vi "Prova NPSH.vi"(7 "Tipo motore pompa":enum16{"Monofase", "Trifase"}(ring), 8 "Array % valvole":dbl[][](array[numeric]), 9 "Manuale F\\auto T":bool=TRUE, 11 "input cluster":T1={"Coefficenti P2"={"Af"=0.0, "Bf"=0.0, "Cf"=0.0, "Df"=0.0, "Ef"=0.0, "Ff"=0.0, "Gf"=0.0, "Hf"=0.0, "Jf"=0.0, "Kf"=0.0, "If"=0.0, "Ar"=0.0, "Br"=0.0, "Cr"=0.0, "Dr"=0.0, "Er"=0.0, "Fr"=0.0, "Gr"=0.0, "Hr"=0.0, "Jr"=0.0, "Kr"=0.0, "Ir"=0.0}, "Cluster settaggi wattmetro"={"Wattmetro"=enum."WT230", "Alimentazione"=enum."Radio Selection 1"}, "CALCOLO POTENZA MECCANICA?"=FALSE, "SET RPM"=0.0, "SET TEMP"=0.0, "IMPOSTAZIONI INGRESSI UL"={"SALVA"=FALSE, "CARICA"=FALSE, "APPLICA"=FALSE, "Q1"={"Range"=0.0, "Offset"=0.0, "Medie"=0}, "Q2"={"Range"=0.0, "Offset"=0.0, "Medie"=0}, "Q3"={"Range"=0.0, "Offset"=0.0, "Medie"=0}, "P1"={"Range"=0.0, "Offset"=0.0, "Medie"=0}, "P2"={"Range"=0.0, "Offset"=0.0, "Medie"=0}, "P3"={"Range"=0.0, "Offset"=0.0, "Medie"=0}, "N"={"Range"=0.0, "Offset"=0.0, "Medie"=0}, "Tq"={"Range"=0.0, "Offset"=0.0, "Medie"=0}, "T"={"Range"=0.0, "Offset"=0.0, "Medie"=0}, "PORTATA PRINCIPALE"=0, "PORTATA SECONDARIA"=0, "PRESSIONE ASPIRAZIONE"=0, "PRESSIONE MANDATA"=0, "RPM"=0, "differenziale?"=FALSE}, "IMPOSTAZIONI INGRESSI NM"={"SALVA"=FALSE, "CARICA"=FALSE, "APPLICA"=FALSE, "Q1"={"Range"=0.0, "Offset"=0.0, "Medie"=0}, "Q2"={"Range"=0.0, "Offset"=0.0, "Medie"=0}, "Q3"={"Range"=0.0, "Offset"=0.0, "Medie"=0}, "Q4"={"Range"=0.0, "Offset"=0.0, "Medie"=0}, "Q5"={"Range"=0.0, "Offset"=0.0, "Medie"=0}, "Q6"={"Range"=0.0, "Offset"=0.0, "Medie"=0}, "Q7"={"Range"=0.0, "Offset"=0.0, "Medie"=0}, "Q8"={"Range"=0.0, "Offset"=0.0, "Medie"=0}, "Q9"={"Range"=0.0, "Offset"=0.0, "Medie"=0}, "Q10"={"Range"=0.0, "Offset"=0.0, "Medie"=0}, "P1"={"Range"=0.0, "Offset"=0.0, "Medie"=0}, "P2"={"Range"=0.0, "Offset"=0.0, "Medie"=0}, "P3"={"Range"=0.0, "Offset"=0.0, "Medie"=0}, "P4"={"Range"=0.0, "Offset"=0.0, "Medie"=0}, "P5"={"Range"=0.0, "Offset"=0.0, "Medie"=0}, "P6"={"Range"=0.0, "Offset"=0.0, "Medie"=0}, "P7"={"Range"=0.0, "Offset"=0.0, "Medie"=0}, "P8"={"Range"=0.0, "Offset"=0.0, "Medie"=0}, "P9"={"Range"=0.0, "Offset"=0.0, "Medie"=0}, "P10"={"Range"=0.0, "Offset"=0.0, "Medie"=0}, "N1(T)"={"Range"=0.0, "Offset"=0.0, "Medie"=0}, "N2(T)"={"Range"=0.0, "Offset"=0.0, "Medie"=0}, "N3(T)"={"Range"=0.0, "Offset"=0.0, "Medie"=0}, "Tq1"={"Range"=0.0, "Offset"=0.0, "Medie"=0}, "Tq2"={"Range"=0.0, "Offset"=0.0, "Medie"=0}, "Tq3"={"Range"=0.0, "Offset"=0.0, "Medie"=0}, "RM1"={"Range"=0.0, "Offset"=0.0, "Medie"=0}, "RM2"={"Range"=0.0, "Offset"=0.0, "Medie"=0}, "RM3"={"Range"=0.0, "Offset"=0.0, "Medie"=0}, "T1"={"Range"=0.0, "Offset"=0.0, "Medie"=0}, "T2"={"Range"=0.0, "Offset"=0.0, "Medie"=0}, "T3"={"Range"=0.0, "Offset"=0.0, "Medie"=0}, "T4"={"Range"=0.0, "Offset"=0.0, "Medie"=0}, "T5"={"Range"=0.0, "Offset"=0.0, "Medie"=0}, "T6"={"Range"=0.0, "Offset"=0.0, "Medie"=0}, "T7"={"Range"=0.0, "Offset"=0.0, "Medie"=0}, "T8"={"Range"=0.0, "Offset"=0.0, "Medie"=0}, "Liv."={"Range"=0.0, "Offset"=0.0, "Medie"=0}, "Pbar"={"Range"=0.0, "Offset"=0.0, "Medie"=0}, "PORTATA\nPRINCIPALE"=0, "PORTATA\nSECONDARIA"=0, "PRESSIONE\nASPIRAZIONE"=0, "PRESSIONE\nMANDATA"=0, "RPM"=0, "differenziale?"=FALSE}, "Costanti collaudo"={"P [bar]"=0.0, "T amb. [°C]"=0.0, "Umidità [%]"=0.0}, "Condizione P2"=enum."Radio Selection 1", "Sett T e R"={"Tamb[°C]"=0.0, "Ru-w"=0.0, "Rmarcia"=0.0, "Raux"=0.0, "Ru-w freddo"=0.0, "Rmarcia freddo"=0.0, "Raux freddop"=0.0, "TC1"=0.0, "TC2"=0.0, "TC3"=0.0, "TC4"=0.0, "TC5"=0.0, "TC6"=0.0, "TC7"=0.0, "TC8"=0.0, "TC9"=0.0}, "Array linee"=[{"portata"=0, "Hasp"=0, "Hmand"=1, "Torsiometro"=0, "rpm"=0, "Hdiff?"=FALSE, "T amb"=0, "Indici valvole"=[0, 1], "Nome"="Elettropompa", "Sommersa?"=FALSE}, {"portata"=1, "Hasp"=0, "Hmand"=0, "Torsiometro"=0, "rpm"=0, "Hdiff?"=FALSE, "T amb"=0, "Indici valvole"=[0, 1], "Nome"="Sommersa", "Sommersa?"=TRUE}], "Array valvole linee avvio/fermata"=[], "Linea selezionata"=0.0} {"IMPOSTAZIONI INGRESSI NM"."T8"."Medie" min=1 step=1; "IMPOSTAZIONI INGRESSI NM"."T7"."Medie" min=1 step=1; "IMPOSTAZIONI INGRESSI NM"."T6"."Medie" min=1 step=1; "IMPOSTAZIONI INGRESSI NM"."T5"."Medie" min=1 step=1; "IMPOSTAZIONI INGRESSI NM"."T4"."Medie" min=1 step=1; "IMPOSTAZIONI INGRESSI NM"."T3"."Medie" min=1 step=1; "IMPOSTAZIONI INGRESSI NM"."RM3"."Medie" min=1 step=1; "IMPOSTAZIONI INGRESSI NM"."Tq3"."Medie" min=1 step=1; "IMPOSTAZIONI INGRESSI NM"."Tq2"."Medie" min=1 step=1; "IMPOSTAZIONI INGRESSI NM"."N3(T)"."Medie" min=1 step=1; "IMPOSTAZIONI INGRESSI NM"."N2(T)"."Medie" min=1 step=1; "IMPOSTAZIONI INGRESSI NM"."P10"."Medie" min=1 step=1; "IMPOSTAZIONI INGRESSI NM"."P9"."Medie" min=1 step=1; "IMPOSTAZIONI INGRESSI NM"."P8"."Medie" min=1 step=1; "IMPOSTAZIONI INGRESSI NM"."P7"."Medie" min=1 step=1; "IMPOSTAZIONI INGRESSI NM"."P6"."Medie" min=1 step=1; "IMPOSTAZIONI INGRESSI NM"."P5"."Medie" min=1 step=1; "IMPOSTAZIONI INGRESSI NM"."Q10"."Medie" min=1 step=1; "IMPOSTAZIONI INGRESSI NM"."Q9"."Medie" min=1 step=1; "IMPOSTAZIONI INGRESSI NM"."Q8"."Medie" min=1 step=1; "IMPOSTAZIONI INGRESSI NM"."Q7"."Medie" min=1 step=1; "IMPOSTAZIONI INGRESSI NM"."Q6"."Medie" min=1 step=1; "IMPOSTAZIONI INGRESSI NM"."Q5"."Medie" min=1 step=1; "IMPOSTAZIONI INGRESSI NM"."Pbar"."Medie" min=1 step=1; "IMPOSTAZIONI INGRESSI NM"."Liv."."Medie" min=1 step=1; "IMPOSTAZIONI INGRESSI NM"."RM2"."Medie" min=1 step=1; "IMPOSTAZIONI INGRESSI NM"."RM1"."Medie" min=1 step=1; "IMPOSTAZIONI INGRESSI NM"."T2"."Medie" min=1 step=1; "IMPOSTAZIONI INGRESSI NM"."P4"."Medie" min=1 step=1; "IMPOSTAZIONI INGRESSI NM"."Q4"."Medie" min=1 step=1; "IMPOSTAZIONI INGRESSI NM"."RPM" items=["TESTO", "TORSIOMETRO", "OTTICA"]; "IMPOSTAZIONI INGRESSI NM"."PRESSIONE\nMANDATA" items=["P1", "P2", "P3", "P4"]; "IMPOSTAZIONI INGRESSI NM"."PRESSIONE\nASPIRAZIONE" items=["P1", "P2", "P3", "P4"]; "IMPOSTAZIONI INGRESSI NM"."PORTATA\nSECONDARIA" items=["Q1", "Q2", "Q3", "Q4"]; "IMPOSTAZIONI INGRESSI NM"."PORTATA\nPRINCIPALE" items=["LINEA ELETTROPOMPA", "LINEA SOMMERSA"]; "IMPOSTAZIONI INGRESSI NM"."T1"."Medie" min=1 step=1; "IMPOSTAZIONI INGRESSI NM"."Tq1"."Medie" min=1 step=1; "IMPOSTAZIONI INGRESSI NM"."N1(T)"."Medie" min=1 step=1; "IMPOSTAZIONI INGRESSI NM"."P3"."Medie" min=1 step=1; "IMPOSTAZIONI INGRESSI NM"."P2"."Medie" min=1 step=1; "IMPOSTAZIONI INGRESSI NM"."P1"."Medie" min=1 step=1; "IMPOSTAZIONI INGRESSI NM"."Q3"."Medie" min=1 step=1; "IMPOSTAZIONI INGRESSI NM"."Q2"."Medie" min=1 step=1; "IMPOSTAZIONI INGRESSI NM"."Q1"."Medie" min=1 step=1; "IMPOSTAZIONI INGRESSI UL"."RPM" items=["TESTO", "TORSIOMETRO", "OTTICA"]; "IMPOSTAZIONI INGRESSI UL"."PRESSIONE MANDATA" items=["P1", "P2", "P3"]; "IMPOSTAZIONI INGRESSI UL"."PRESSIONE ASPIRAZIONE" items=["P1", "P2", "P3"]; "IMPOSTAZIONI INGRESSI UL"."PORTATA SECONDARIA" items=["Q1", "Q2", "Q3"]; "IMPOSTAZIONI INGRESSI UL"."PORTATA PRINCIPALE" items=["Q1", "Q2", "Q3"]; "IMPOSTAZIONI INGRESSI UL"."T"."Medie" min=1 step=1; "IMPOSTAZIONI INGRESSI UL"."Tq"."Medie" min=1 step=1; "IMPOSTAZIONI INGRESSI UL"."N"."Medie" min=1 step=1; "IMPOSTAZIONI INGRESSI UL"."P3"."Medie" min=1 step=1; "IMPOSTAZIONI INGRESSI UL"."P2"."Medie" min=1 step=1; "IMPOSTAZIONI INGRESSI UL"."P1"."Medie" min=1 step=1; "IMPOSTAZIONI INGRESSI UL"."Q3"."Medie" min=1 step=1; "IMPOSTAZIONI INGRESSI UL"."Q2"."Medie" min=1 step=1; "IMPOSTAZIONI INGRESSI UL"."Q1"."Medie" min=1 step=1}) -> ()   [LabVIEW 2016]
uses:
  TypeDef/ALIM SELECTION.ctl
  TypeDef/WT SELECTION.ctl
  TypeDef/SETUP INGRESSO.ctl
  TypeDef/cDAQ Settings UL.ctl
  TypeDef/cDAQ Settings NM.ctl
  TypeDef/sett T e R.ctl
  TypeDef/Definizione linea.ctl
  TypeDef/Cluster INFO.ctl
panel:
  in  "Status":refnum<vi>
  # "Freddo"
  # "Regime"
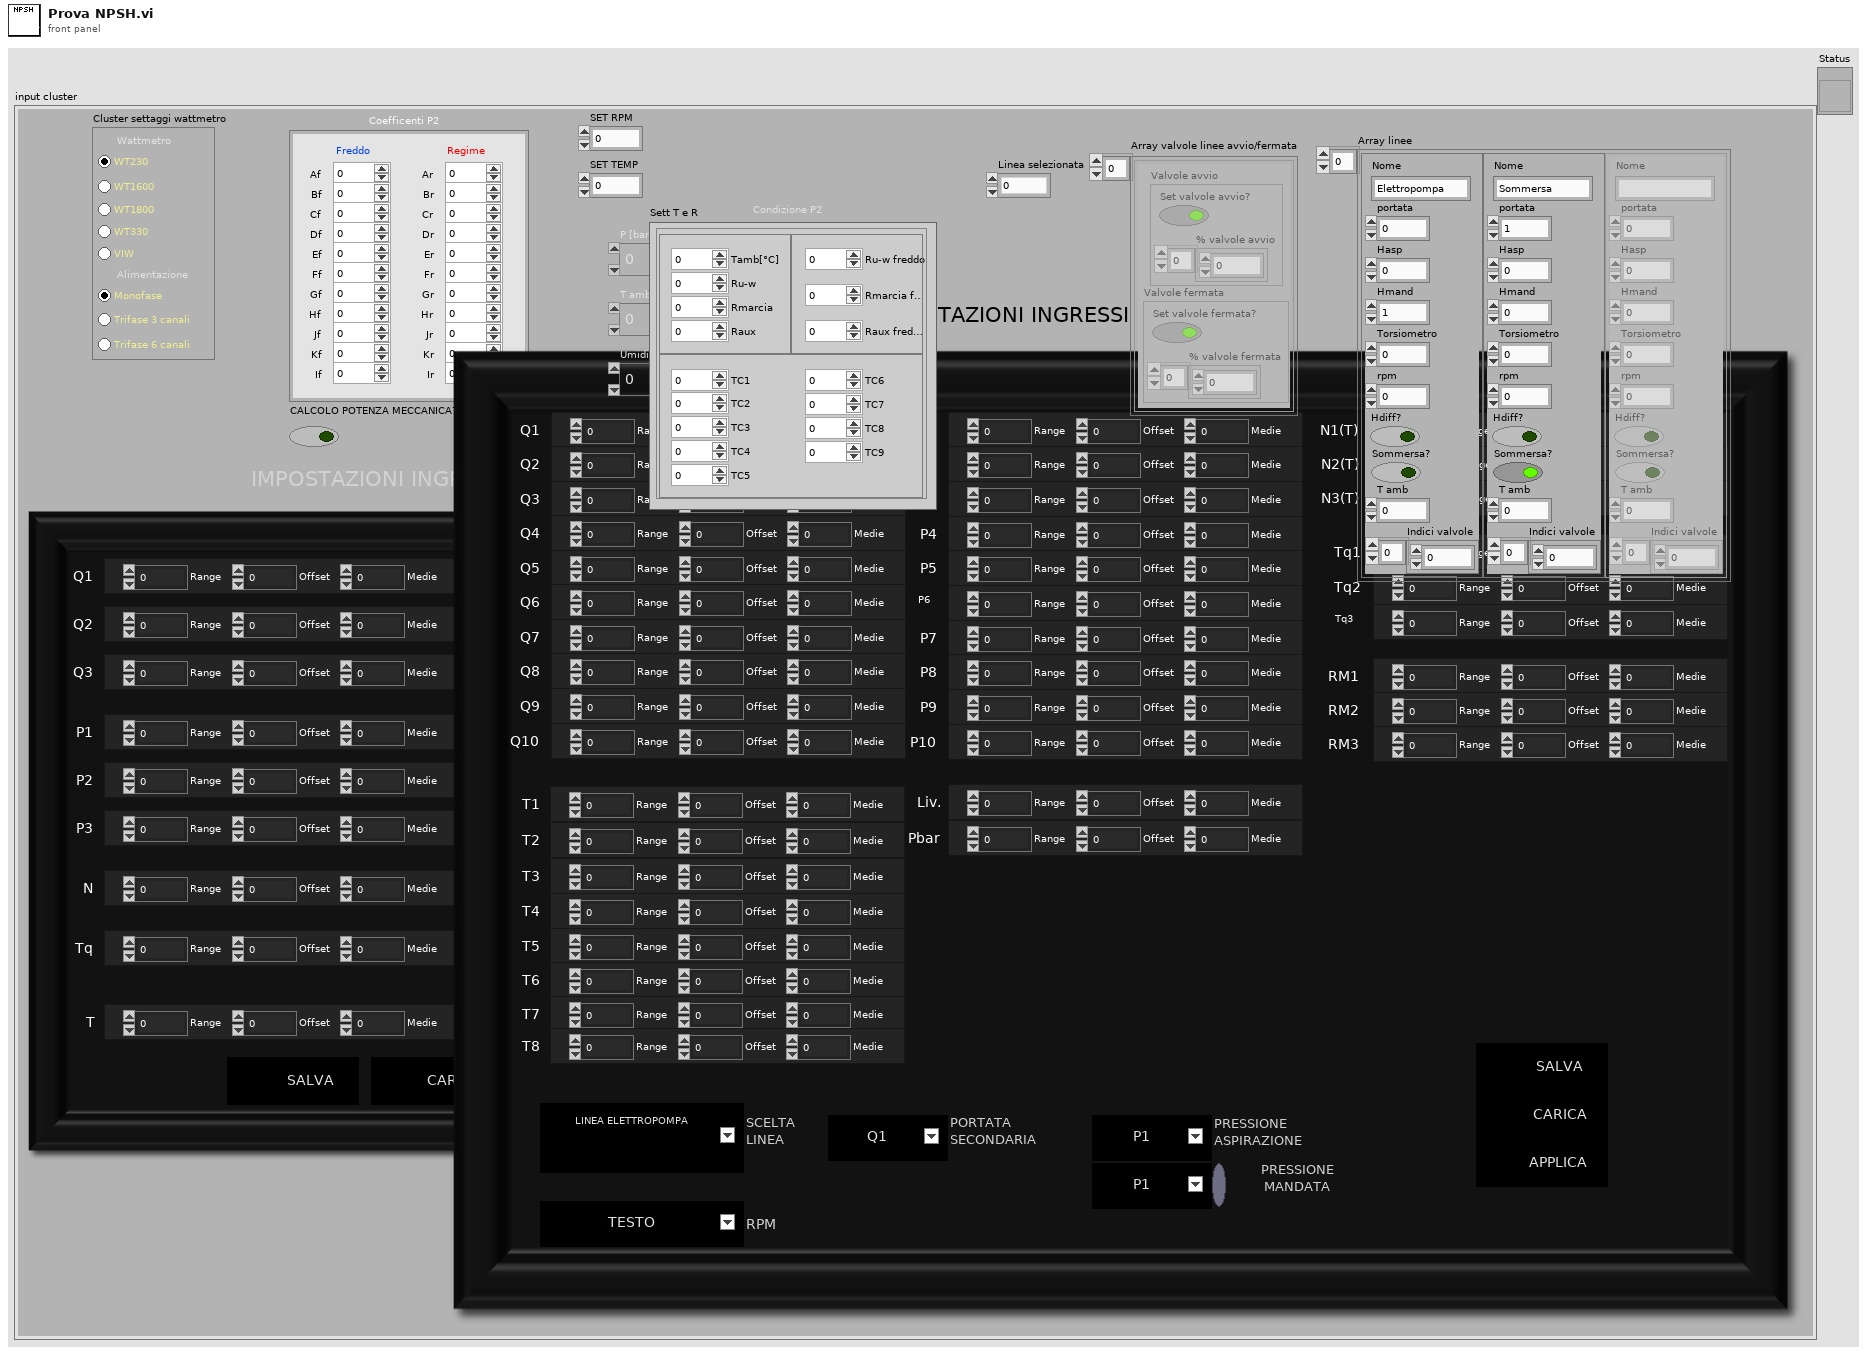
[diagram p1: front panel]
types:
  T1 = typedef "Cluster INFO.ctl" = cluster{"Coefficenti P2":cluster{"Af":dbl, "Bf":dbl, "Cf":dbl, "Df":dbl, "Ef":dbl, "Ff":dbl, "Gf":dbl, "Hf":dbl, "Jf":dbl, "Kf":dbl, "If":dbl, "Ar":dbl, "Br":dbl, "Cr":dbl, "Dr":dbl, "Er":dbl, "Fr":dbl, "Gr":dbl, "Hr":dbl, "Jr":dbl, "Kr":dbl, "Ir":dbl}, "Cluster settaggi wattmetro":cluster{"Wattmetro":T2, "Alimentazione":T3}, "CALCOLO POTENZA MECCANICA?":bool, "SET RPM":dbl, "SET TEMP":dbl, "IMPOSTAZIONI INGRESSI UL":T4, "IMPOSTAZIONI INGRESSI NM":T6, "Costanti collaudo":cluster{"P [bar]":dbl, "T amb. [°C]":dbl, "Umidità [%]":dbl}, "Condizione P2":enum32{"Radio Selection 1", "Radio Selection 2"}, "Sett T e R":T7, "Array linee":T8[], "Array valvole linee avvio/fermata":cluster{"Valvole avvio":cluster{"Set valvole avvio?":bool, "% valvole avvio":dbl[]}, "Valvole fermata":cluster{"Set valvole fermata?":bool, "% valvole fermata":dbl[]}}[], "Linea selezionata":dbl}
  T2 = typedef "WT SELECTION.ctl" = enum32{"No Selection", "WT230", "WT1600", "WT1800", "WT330", "VIW"}
  T3 = typedef "ALIM SELECTION.ctl" = enum32{"Radio Selection 1", "Radio Selection 2", "Radio Selection 3"}
  T4 = typedef "cDAQ Settings UL.ctl" = cluster{"SALVA":bool, "CARICA":bool, "APPLICA":bool, "Q1":T5, "Q2":T5, "Q3":T5, "P1":T5, "P2":T5, "P3":T5, "N":T5, "Tq":T5, "T":T5, "PORTATA PRINCIPALE":u16, "PORTATA SECONDARIA":u16, "PRESSIONE ASPIRAZIONE":u16, "PRESSIONE MANDATA":u16, "RPM":u16, "differenziale?":bool}
  T5 = typedef "SETUP INGRESSO.ctl" = cluster{"Range":dbl, "Offset":dbl, "Medie":u8}
  T6 = typedef "cDAQ Settings NM.ctl" = cluster{"SALVA":bool, "CARICA":bool, "APPLICA":bool, "Q1":T5, "Q2":T5, "Q3":T5, "Q4":T5, "Q5":T5, "Q6":T5, "Q7":T5, "Q8":T5, "Q9":T5, "Q10":T5, "P1":T5, "P2":T5, "P3":T5, "P4":T5, "P5":T5, "P6":T5, "P7":T5, "P8":T5, "P9":T5, "P10":T5, "N1(T)":T5, "N2(T)":T5, "N3(T)":T5, "Tq1":T5, "Tq2":T5, "Tq3":T5, "RM1":T5, "RM2":T5, "RM3":T5, "T1":T5, "T2":T5, "T3":T5, "T4":T5, "T5":T5, "T6":T5, "T7":T5, "T8":T5, "Liv.":T5, "Pbar":T5, "PORTATA\nPRINCIPALE":u16, "PORTATA\nSECONDARIA":u16, "PRESSIONE\nASPIRAZIONE":u16, "PRESSIONE\nMANDATA":u16, "RPM":u16, "differenziale?":bool}
  T7 = typedef "sett T e R.ctl" = cluster{"Tamb[°C]":dbl, "Ru-w":dbl, "Rmarcia":dbl, "Raux":dbl, "Ru-w freddo":dbl, "Rmarcia freddo":dbl, "Raux freddop":dbl, "TC1":dbl, "TC2":dbl, "TC3":dbl, "TC4":dbl, "TC5":dbl, "TC6":dbl, "TC7":dbl, "TC8":dbl, "TC9":dbl}
  T8 = typedef "Definizione linea.ctl" = cluster{"portata":i32, "Hasp":i32, "Hmand":i32, "Torsiometro":i32, "rpm":i32, "Hdiff?":bool, "T amb":i32, "Indici valvole":i16[], "Nome":string, "Sommersa?":bool}
  T9 = cluster{"Valvole avvio":cluster{"Set valvole avvio?":bool, "% valvole avvio":dbl[]}, "Valvole fermata":cluster{"Set valvole fermata?":bool, "% valvole fermata":dbl[]}}[]
  T10 = cluster{"Valvole avvio":cluster{"Set valvole avvio?":bool, "% valvole avvio":dbl[]}, "Valvole fermata":cluster{"Set valvole fermata?":bool, "% valvole fermata":dbl[]}}
  T11 = cluster{"Set valvole avvio?":bool, "% valvole avvio":dbl[]}
  T12 = cluster{"Set valvole fermata?":bool, "% valvole fermata":dbl[]}
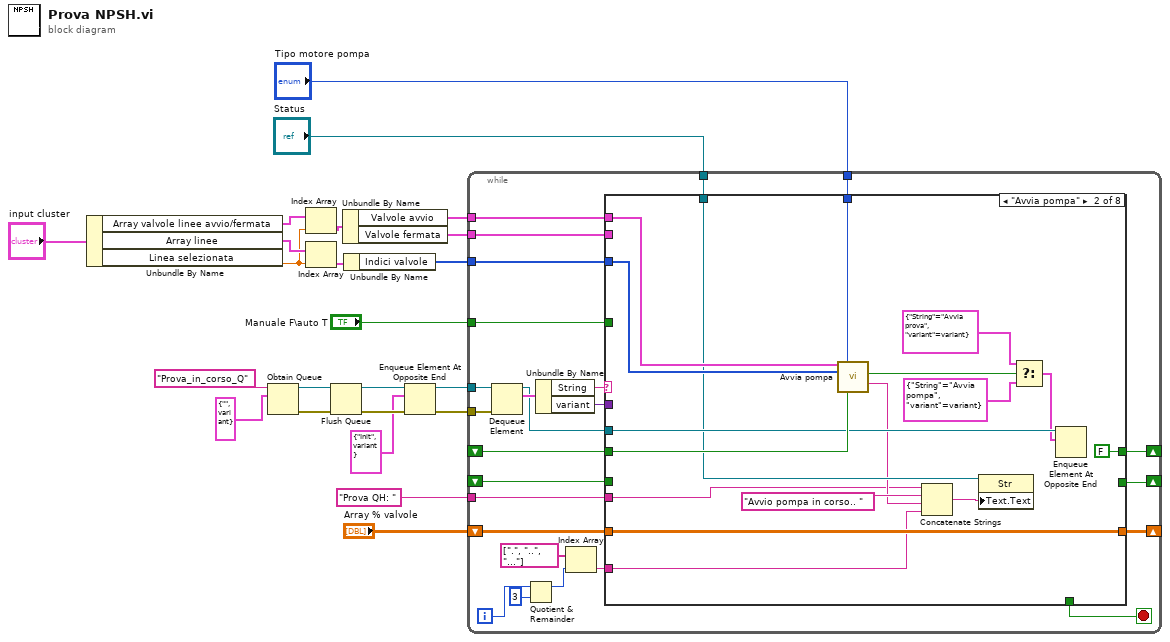
[diagram p0: block diagram]
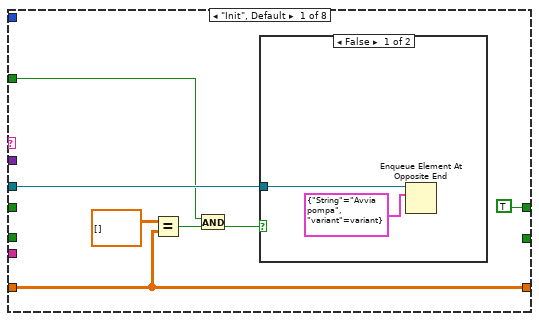
[diagram p2: hidden frame]
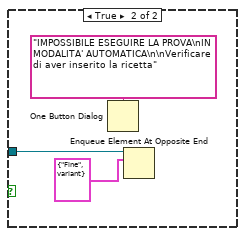
[diagram p3: hidden frame]
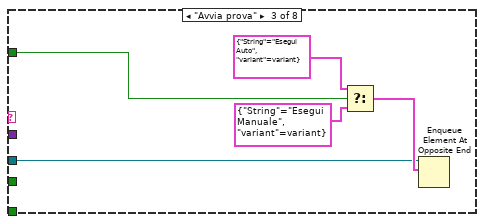
[diagram p4: hidden frame]
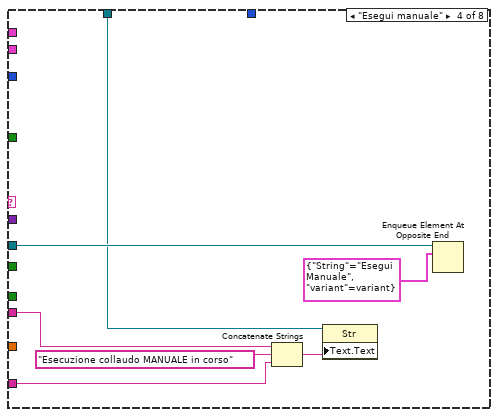
[diagram p5: hidden frame]
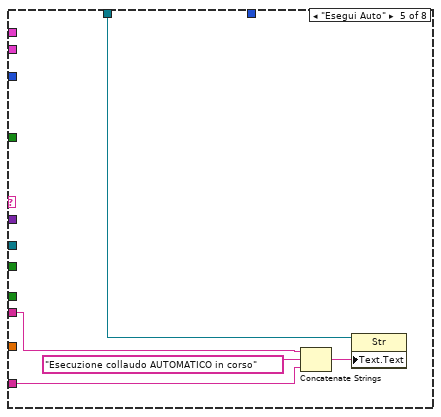
[diagram p6: hidden frame]
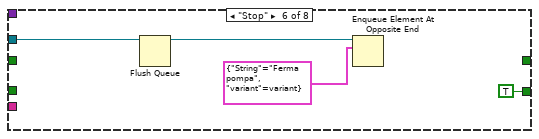
[diagram p7: hidden frame]
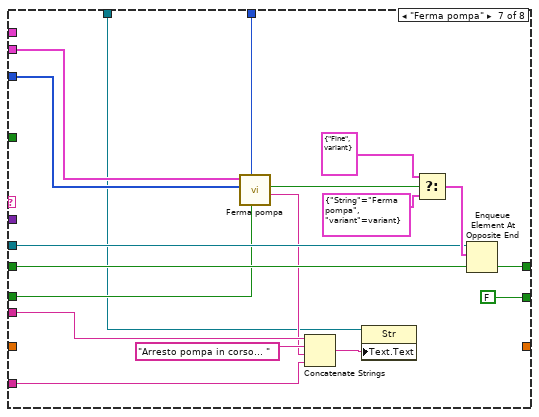
[diagram p8: hidden frame]
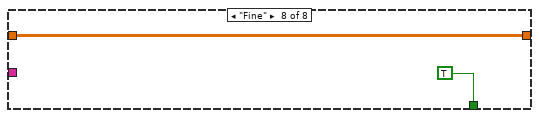
[diagram p9: hidden frame]
diagram:
  n1 = Unbundle By Name("input cluster") -> ("Array valvole linee avvio/fermata"=w9:T9, "Array linee"=w11:T8[], "Linea selezionata"=w8:dbl)
  n2 = Obtain Queue(name (unnamed)="Prova_in_corso_Q" ("Queue Name"), element data type=cluster{"String":string, "variant":variant} {"String"="", "variant"=variant} ("element")) -> (queue out=w17:refnum<queue>, error out=w16:errorcluster)  [unwired: 3 in, 1 out]
  n3 = Index Array(array=w9, index=w8) -> (element=w7:T10)
  n4 = Index Array(array=w11, index=w8) -> (element=w10:T8)
  n5 = Flush Queue(queue=w17, error in (no error)=w16) -> (queue out=w21:refnum<queue>, error out=w20:errorcluster)  [unwired: 1 out]
  n6 = Unbundle By Name(w7) -> ("Valvole avvio"=w5:T11, "Valvole fermata"=w4:T12)
  n7 = Unbundle By Name(w10) -> ("Indici valvole"=w3:i16[])
  n8 = Enqueue Element At Opposite End(queue=w21, element=cluster{"String":string, "variant":variant} {"String"="Init", "variant"=variant}, error in (no error)=w20) -> (queue out=w23:refnum<queue>, error out=w22:errorcluster)  [unwired: 1 in, 1 out]
  n9 = while {
    tunnel: w23 -> [w48]
    tunnel: w22 -> [w47]
    tunnel: "Manuale F\\auto T" -> [w43]
    shift-right: [w42] -> _
    shift-left: "Array % valvole" -> [w41]
    shift-right: [w39] -> _
    shift-left: _ -> [w38]
    tunnel: w5 -> [w37]
    tunnel: "Tipo motore pompa" -> [w36]
    tunnel: w4 -> [w35]
    shift-right: [w34] -> _
    shift-left: _ -> [w33]
    tunnel: w3 -> [w32]
    tunnel: "Status" -> [w31]
    tunnel: "Prova QH: " ("Text.Text") -> [w29]
    i -> [w25]
    stop <- w30 stop-if-true
    n10 = Dequeue Element(queue=w48, error in (no error)=w47) -> (queue out=w40:refnum<queue>, element=w46:cluster{"String":string, "variant":variant})  [unwired: 1 in, 2 out]
    n11 = Quotient & Remainder(x=w25, y=3) -> (x-y*floor(x/y)=w28:i32)  [unwired: 1 out]
    n12 = Unbundle By Name(w46) -> ("String"=w45:string, "variant"=w44:variant)
    n13 = Index Array(array=string[] [".", "..", "..."], index=w28) -> (element=w24:string)
    n14 = case shown="\"Avvia pompa\"" w45 {
      tunnel: w44 -> [_ _ _ _ _ _ _ _]
      tunnel: w43 -> [w49 _ w78 _ _ _ _ _]
      tunnel: [w55 w70 _ _ _ _ _ w117] -> w42
      tunnel: w41 -> [w55 w70 _ _ _ _ _ w117]
      tunnel: w40 -> [w52 w75 w79 w88 _ w98 w108 _]
      tunnel: [TRUE FALSE _ _ _ _ w113 _] -> w39
      tunnel: w38 -> [_ w77 _ _ _ _ w113 _]
      tunnel: w37 -> [_ w68 _ _ _ _ _ _]
      tunnel: w36 -> [_ w69 _ _ _ _ w114 _]
      tunnel: w35 -> [_ _ _ _ _ _ w106 _]
      tunnel: [_ _ _ _ _ TRUE FALSE _] -> w34
      tunnel: w33 -> [_ _ _ _ _ _ w107 _]
      tunnel: w32 -> [_ w67 _ _ _ _ w105 _]
      tunnel: w31 -> [_ w66 _ w87 w92 _ w99 _]
      tunnel: [_ _ _ _ _ _ _ TRUE] -> w30
      tunnel: w29 -> [_ w62 _ w86 w91 _ w103 _]
      tunnel: w24 -> [_ w61 _ w83 w90 _ w100 _]
      frame "Init", Default {
        n15 = Equal?(x=dbl[][] [], y=w55) -> (x = y?=w53:bool)
        n16 = And(x=w49, y=w53) -> (x .and. y?=w50:bool)
        n17 = case shown="False" w50 {
          tunnel: w52 -> [w56 w59]
          frame False {
            n18 = Enqueue Element At Opposite End(queue=w56, element=cluster{"String":string, "variant":variant} {"String"="Avvia pompa", "variant"=variant}) -> ()  [unwired: 2 in, 3 out]
          }
          frame True {
            n19 = One Button Dialog(message="IMPOSSIBILE ESEGUIRE LA PROVA\nIN MODALITA' AUTOMATICA\n\nVerificare di aver inserito la ricetta") -> ()  [unwired: 1 in, 1 out]
            n20 = Enqueue Element At Opposite End(queue=w59, element=cluster{"String":string, "variant":variant} {"String"="Fine", "variant"=variant}) -> ()  [unwired: 2 in, 3 out]
          }
        }
      }
      frame "Avvia pompa" {
        n21 = call "Avvia pompa.vi"("Valvole avvio"=w68, "Tipo motore pompa"=w69, "Indici valvole linea"=w67, "Reset avvio"=w77) -> ("Fine Avvio"=w74:bool, "stato"=w63:string)  [unwired: 10 in]
        n22 = Concatenate Strings(w62, "Avvio pompa in corso.. " ("Text.Text"), w63, w61) -> (w64:string)
        n23 = property class="Str"(reference=w66, "Text.Text"=w64) -> ()  [unwired: 1 in, 2 out]
        n24 = Select(t=cluster{"String":string, "variant":variant} {"String"="Avvia prova", "variant"=variant} ("element"), s=w74, f=cluster{"String":string, "variant":variant} {"String"="Avvia pompa", "variant"=variant} ("element")) -> (s? t:f=w72:cluster{"String":string, "variant":variant})
        n25 = Enqueue Element At Opposite End(queue=w75, element=w72) -> ()  [unwired: 2 in, 3 out]
      }
      frame "Avvia prova" {
        n26 = Select(t=cluster{"String":string, "variant":variant} {"String"="Esegui Auto", "variant"=variant} ("element"), s=w78, f=cluster{"String":string, "variant":variant} {"String"="Esegui Manuale", "variant"=variant} ("element")) -> (s? t:f=w81:cluster{"String":string, "variant":variant})
        n27 = Enqueue Element At Opposite End(queue=w79, element=w81) -> ()  [unwired: 2 in, 3 out]
      }
      frame "Esegui manuale" {
        n28 = Concatenate Strings(w86, "Esecuzione collaudo MANUALE in corso" ("string"), w83) -> (w85:string)
        n29 = property class="Str"(reference=w87, "Text.Text"=w85) -> ()  [unwired: 1 in, 2 out]
        n30 = Enqueue Element At Opposite End(queue=w88, element=cluster{"String":string, "variant":variant} {"String"="Esegui Manuale", "variant"=variant}) -> ()  [unwired: 2 in, 3 out]
      }
      frame "Esegui Auto" {
        n31 = Concatenate Strings(w91, "Esecuzione collaudo AUTOMATICO in corso" ("string"), w90) -> (w94:string)
        n32 = property class="Str"(reference=w92, "Text.Text"=w94) -> ()  [unwired: 1 in, 2 out]
      }
      frame "Stop" {
        n33 = Flush Queue(queue=w98) -> (queue out=w96:refnum<queue>)  [unwired: 1 in, 2 out]
        n34 = Enqueue Element At Opposite End(queue=w96, element=cluster{"String":string, "variant":variant} {"String"="Ferma pompa", "variant"=variant}) -> ()  [unwired: 2 in, 3 out]
      }
      frame "Ferma pompa" {
        n35 = call "Ferma pompa.vi"("Reset fermata"=w107, "Tipo motore pompa"=w114, "Indici valvole linea"=w105, "Valvole fermata"=w106) -> ("stato"=w101:string, "Fine Fermata"=w109:bool)  [unwired: 6 in]
        n36 = Concatenate Strings(w103, "Arresto pompa in corso... " ("string"), w101, w100) -> (w104:string)
        n37 = property class="Str"(reference=w99, "Text.Text"=w104) -> ()  [unwired: 1 in, 2 out]
        n38 = Select(t=cluster{"String":string, "variant":variant} {"String"="Fine", "variant"=variant} ("element"), s=w109, f=cluster{"String":string, "variant":variant} {"String"="Ferma pompa", "variant"=variant} ("element")) -> (s? t:f=w111:cluster{"String":string, "variant":variant})
        n39 = Enqueue Element At Opposite End(queue=w108, element=w111) -> ()  [unwired: 2 in, 3 out]
      }
      frame "Fine" {
      }
    }
  }
